vi "Seq Dialog Set Digital Output.vi"(8 "Segment Data":T2) -> (0 "Step Hisitory":string[](array[string]), 2 "Segment Data 2":T2)   [LabVIEW 2018]
uses:
  type defs/EOL Global Digital Output Control.ctl
  type defs/Sequence Info.ctl
  type defs/EOL Global Digital Output Cluster Control.ctl
panel:
  in  "Boolean":bool
  in  "Digital Input":T1
  out "Name":string="Pre Run Station - Glass - Vent Open"
  in  "Description":string
  in  "Save":bool
  in  "Cancel":bool
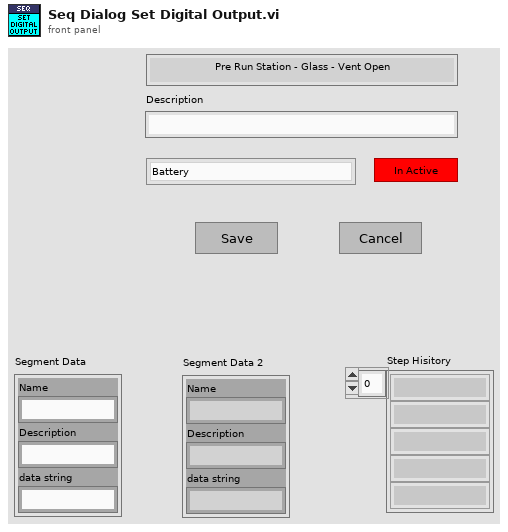
[diagram p1: front panel]
types:
  T1 = typedef "EOL Global Digital Output Control.ctl" = enum16{"Battery", "IGN High", "IGN Low", "LIN", "CAN", "Switch 1", "Switch 2", "Switch 3", "Switch 4", "Switch 5", "Switch 6", "Glass Analog Switch 1", "Glass Analog Switch 2", "Glass Analog Switch 3", "Glass Analog Switch 4", "Sunshade Analog Switch 1", "Sunshade Analog Switch 2", "Sunshade Analog Switch 3", "Sunshade Analog Switch 4", "Glass Motor Relay 1", "Glass Motor Relay 2", "Sunshade Motor Relay 1", "Sunshade Motor Relay 2"}
  T2 = typedef "Sequence Info.ctl" = cluster{"Name":string, "Description":string, "data string":string}
  T3 = typedef "EOL Global Digital Output Cluster Control.ctl" = cluster{"Status":bool, "Global DO Ch":T1}
  T4 = cluster{"Segment Data":T2, "Old Data":string, "New Data":string, "Global Digital Input Cluster":T3}
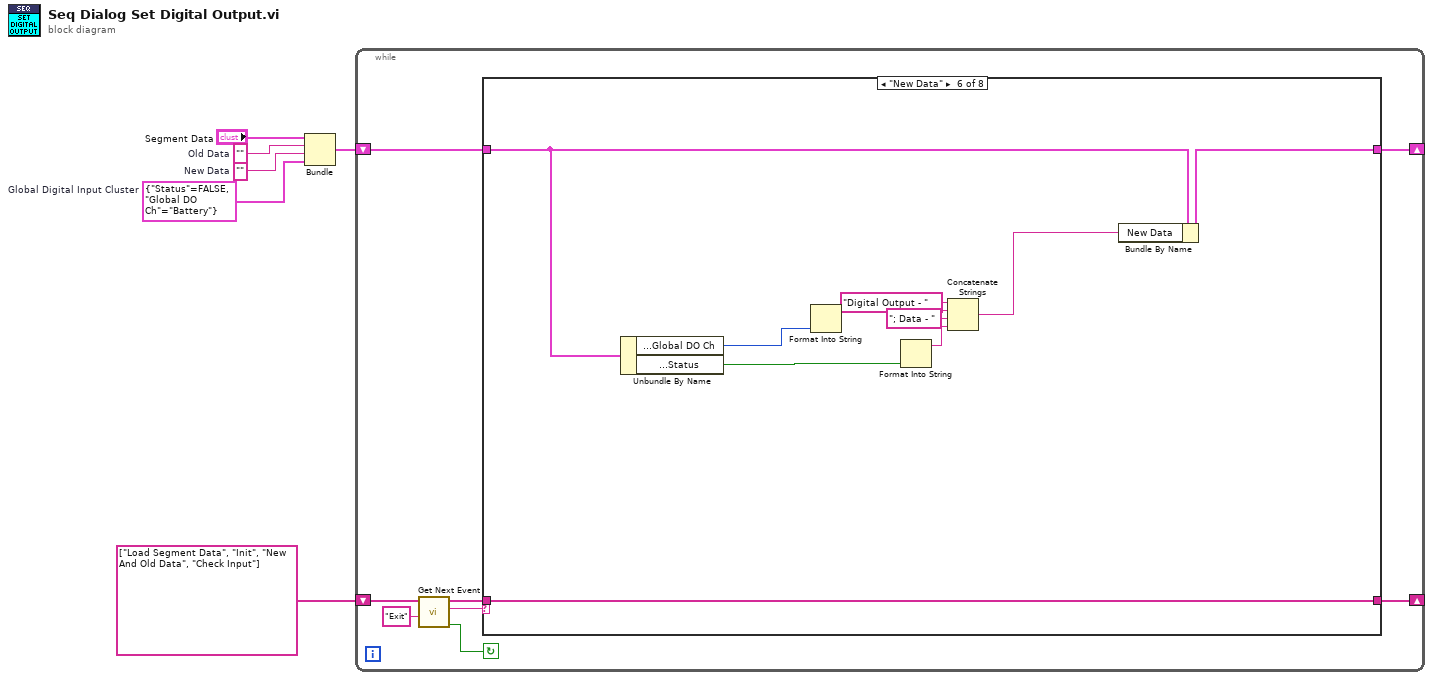
[diagram p0: block diagram]
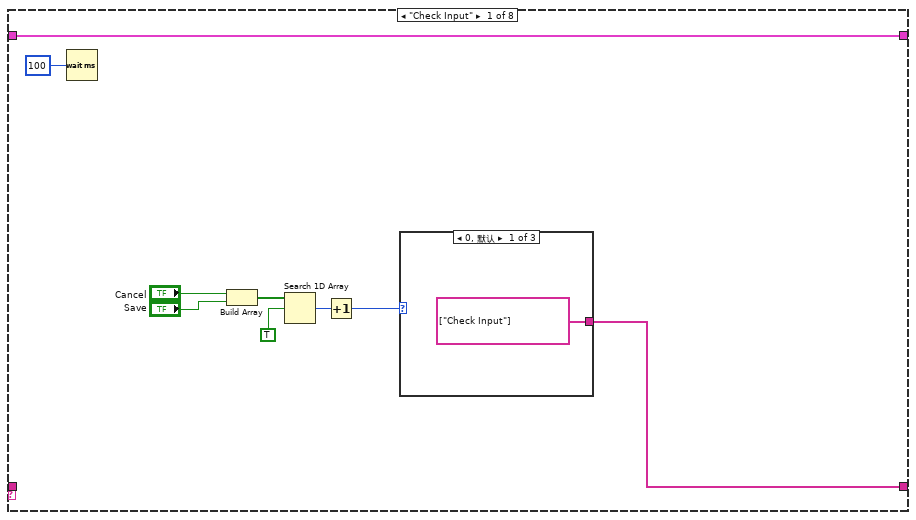
[diagram p2: hidden frame]
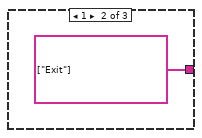
[diagram p3: hidden frame]
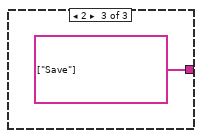
[diagram p4: hidden frame]
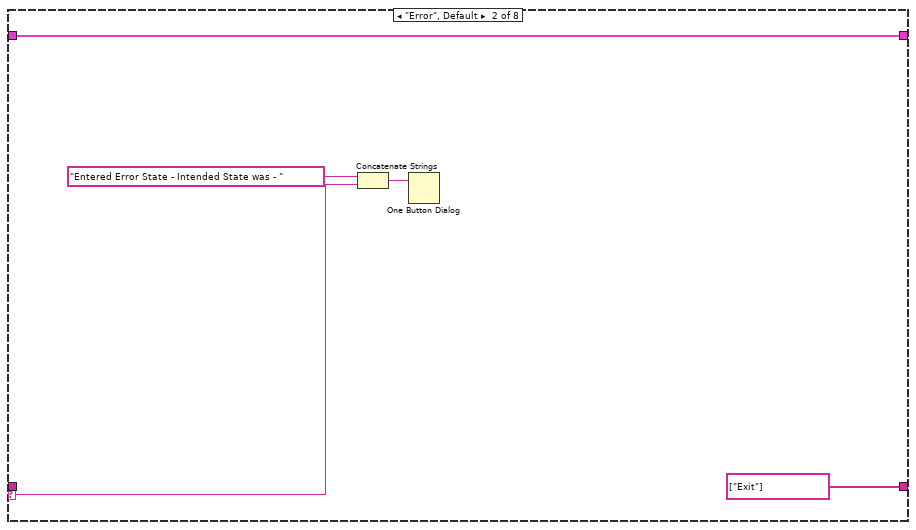
[diagram p5: hidden frame]
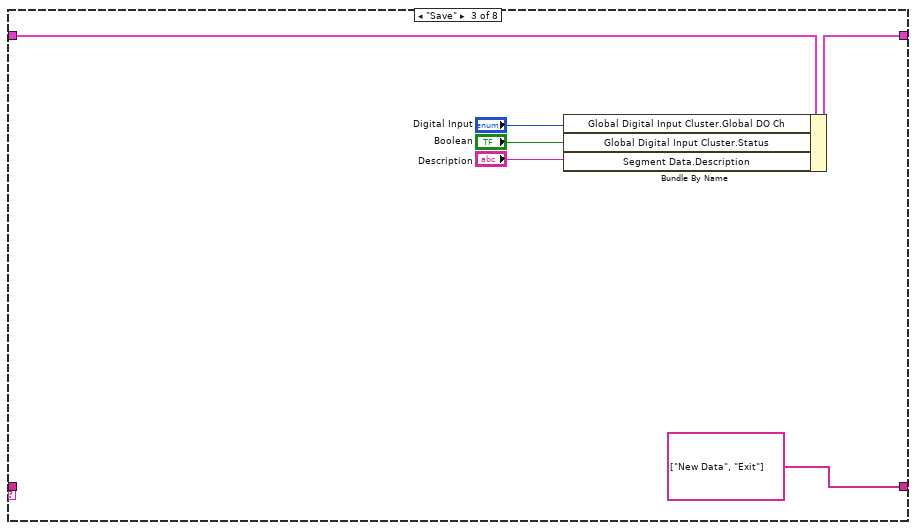
[diagram p6: hidden frame]
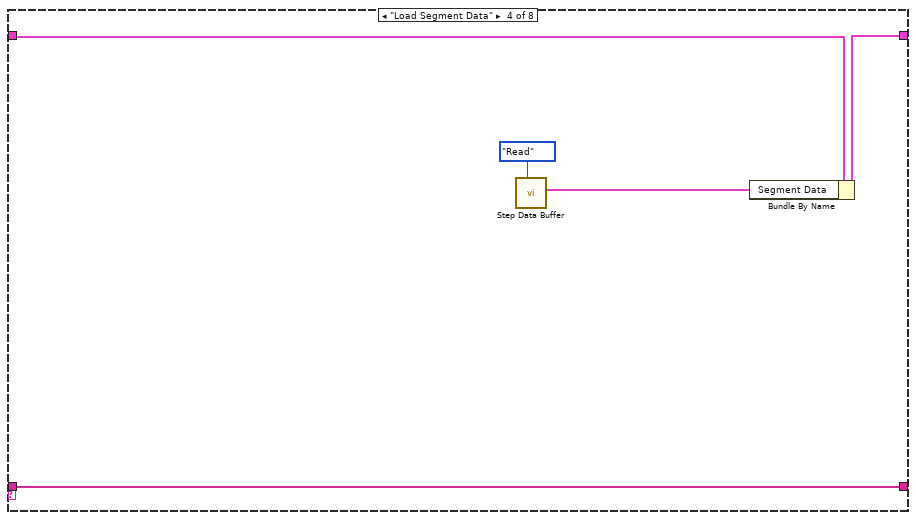
[diagram p7: hidden frame]
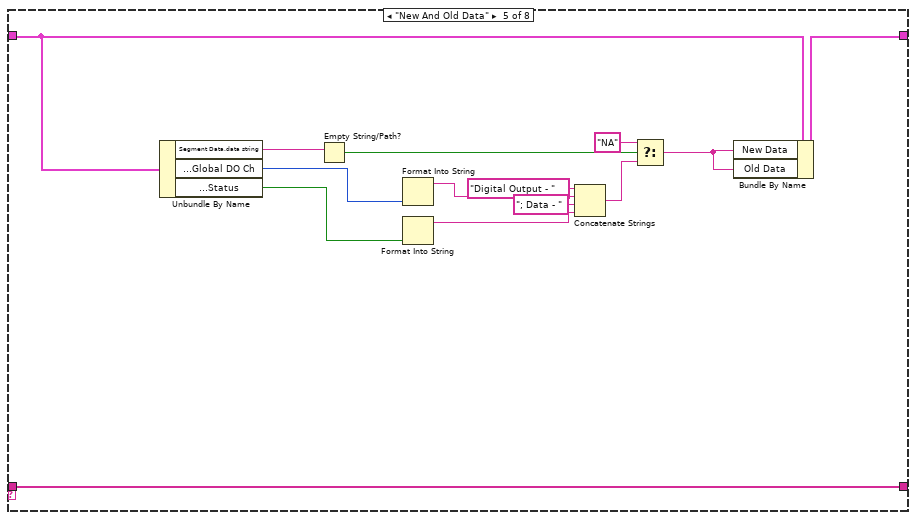
[diagram p8: hidden frame]
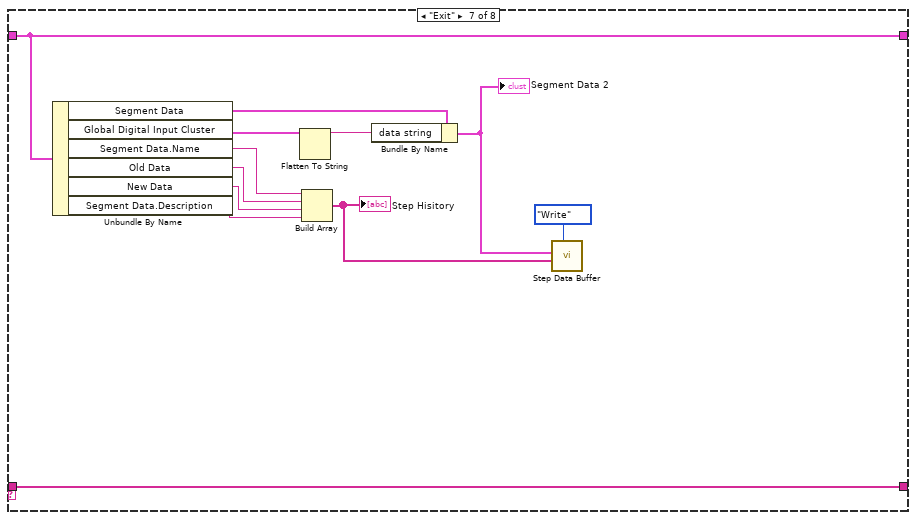
[diagram p9: hidden frame]
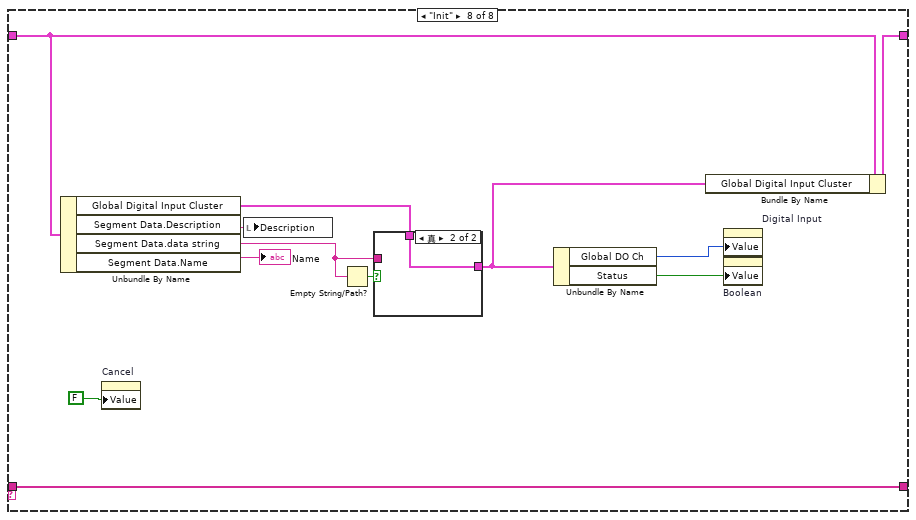
[diagram p10: hidden frame]
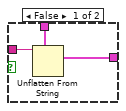
[diagram p11: hidden frame]
diagram:
  w1 = T3 {"Status"=FALSE, "Global DO Ch"=enum."Battery"}  # Global Digital Input Cluster
  w3 = ""  # New Data
  w4 = ""  # Old Data
  n1 = Bundle("Segment Data"="Segment Data", "Old Data"=w4, "New Data"=w3, "Global Digital Input Cluster"=w1) -> (w6:T4)  [unwired: 1 in]
  n2 = while {
    shift-right: [w12] -> _
    shift-left: string[] ["Load Segment Data", "Init", "New And Old Data", "Check Input"] ("Event queue out") -> [w11]
    shift-right: [w7] -> _
    shift-left: w6 -> [w8]
    stop <- w10 continue-if-true
    n3 = call "Get Next Event.vi"("Exit Event"="Exit", "event queue in"=w11) -> ("Condition (Exit:F)"=w10:bool, "next event"=w14:string, "event queue out"=w13:string[])  [unwired: 3 in]
    n4 = case shown="\"New Data\"" w14 {
      selector: w14 -> [_ w29 _ _ _ _ _ _]
      tunnel: w13 -> [_ _ _ w38 w50 w66 w78 w90]
      tunnel: [w17 string[] ["Exit"] ("event queue out") string[] ["New Data", "Exit"] ("Event queue out") w38 w50 w66 w78 w90] -> w12
      tunnel: w8 -> [w22 w27 w36 w40 w52 w65 w77 w85]
      tunnel: [w22 w27 w37 w39 w51 w64 w77 w82] -> w7
      frame "Check Input" {
        n5 = Wait (ms)(milliseconds to wait=u32 100) -> ()  [unwired: 1 out]
        n6 = Build Array("Cancel", "Save") -> (w19:bool[])
        n7 = Search 1D Array(1D array=w19, element=TRUE) -> (index of element=w20:i32)  [unwired: 1 in]
        n8 = Increment(x=w20) -> (x+1=w21:i32)
        n9 = case shown="0, 默认" w21 {
          tunnel: [string[] ["Check Input"] ("Events to Insert") string[] ["Exit"] ("Events to Insert") string[] ["Save"] ("Events to Insert")] -> w17
          frame 0, Default {
          }
          frame 1 {
          }
          frame 2 {
          }
        }
      }
      frame "Error", Default {
        n10 = Concatenate Strings("Entered Error State - Intended State was - " ("string"), w29) -> (w31:string)
        n11 = One Button Dialog(message=w31) -> ()  [unwired: 1 in, 1 out]
      }
      frame "Save" {
        n12 = Bundle By Name(cluster=w36, "Global Digital Input Cluster.Global DO Ch"="Digital Input", "Global Digital Input Cluster.Status"="Boolean", "Segment Data.Description"="Description") -> (w37:T4)
      }
      frame "Load Segment Data" {
        n13 = call "Step Data Buffer.vi"("Mode"=enum16{"Init", "Read", "Write"}."Read") -> ("Segment Data Out"=w42:T2)  [unwired: 6 in, 4 out]
        n14 = Bundle By Name(cluster=w40, "Segment Data"=w42) -> (w39:T4)
      }
      frame "New And Old Data" {
        n15 = Unbundle By Name(w52) -> ("Segment Data.data string"=w56:string, "Global Digital Input Cluster.Global DO Ch"=w44:T1, "Global Digital Input Cluster.Status"=w46:bool)
        n16 = Empty String/Path?(string/path=w56) -> (empty?=w53:bool)
        n17 = Format Into String(w44) -> (resulting string=w43:string)  [unwired: 3 in, 1 out]
        n18 = Format Into String(w46) -> (resulting string=w45:string)  [unwired: 3 in, 1 out]
        n19 = Concatenate Strings("Digital Output - " ("string"), w43, "; Data - " ("string"), w45) -> (w47:string)
        n20 = Select(t="NA", s=w53, f=w47) -> (s? t:f=w55:string)
        n21 = Bundle By Name(cluster=w52, "New Data"=w55, "Old Data"=w55) -> (w51:T4)
      }
      frame "New Data" {
        n22 = Unbundle By Name(w65) -> ("Global Digital Input Cluster.Global DO Ch"=w58:T1, "Global Digital Input Cluster.Status"=w60:bool)
        n23 = Format Into String(w58) -> (resulting string=w57:string)  [unwired: 3 in, 1 out]
        n24 = Format Into String(w60) -> (resulting string=w59:string)  [unwired: 3 in, 1 out]
        n25 = Concatenate Strings("Digital Output - " ("string"), w57, "; Data - " ("string"), w59) -> (w61:string)
        n26 = Bundle By Name(cluster=w65, "New Data"=w61) -> (w64:T4)
      }
      frame "Exit" {
        n27 = Unbundle By Name(w77) -> ("Segment Data"=w70:T2, "Global Digital Input Cluster"=w68:T3, "Segment Data.Name"=w76:string, "Old Data"=w75:string, "New Data"=w74:string, "Segment Data.Description"=w71:string)
        n28 = Flatten To String(anything=w68) -> (data string=w67:string)  [unwired: 3 in, 2 out]
        n29 = Build Array(w76, w75, w74, w71) -> (w72:string[])
        "Step Hisitory" <- w72
        n30 = Bundle By Name(cluster=w70, "data string"=w67) -> (w69:T2)
        "Segment Data 2" <- w69
        n31 = call "Step Data Buffer.vi"("Mode"=enum16{"Init", "Read", "Write"}."Write", "Step Hisitory In"=w72, "Segment Data In"=w69) -> ()  [unwired: 4 in, 5 out]
      }
      frame "Init" {
        n32 = Unbundle By Name(w85) -> ("Global Digital Input Cluster"=w86:T3, "Segment Data.Description"=w89:string, "Segment Data.data string"=w83:string, "Segment Data.Name"=→"Name":string)
        n33 = property on="Cancel" class="Bool (严格)"("Value"=FALSE ("Cancel")) -> ()  [unwired: 2 in, 2 out]
        n34 = local write "Description"(w89) -> ()
        n35 = Empty String/Path?(string/path=w83) -> (empty?=w84:bool)
        n36 = case shown="真" w84 {
          tunnel: w83 -> [w93 _]
          tunnel: w86 -> [w92 w94]
          tunnel: [w91 w94] -> w80
          frame False {
            n37 = Unflatten From String(type=w92, binary string=w93) -> (value=w91:T3)  [unwired: 3 in, 2 out]
          }
          frame True {
          }
        }
        n38 = Unbundle By Name(w80) -> ("Global DO Ch"=w79:T1, "Status"=w81:bool)
        n39 = Bundle By Name(cluster=w85, "Global Digital Input Cluster"=w80) -> (w82:T4)
        n40 = property on="Digital Input" class="Enum (严格)"("Value"=w79) -> ()  [unwired: 2 in, 2 out]
        n41 = property on="Boolean" class="Bool (严格)"("Value"=w81) -> ()  [unwired: 2 in, 2 out]
      }
    }
  }
